vi "ni579x Validate Clock Configuration.vi"(0 "Register Bus":refnum<class "ni579x Register Bus v1 Host.lvclass">=refnum, 1 "scope":string, 5 "clock source":string(combo), 7 "reference clock source":string(combo), 11 "Error In":errorcluster) -> (4 "Register Bus (out)":refnum<class "ni579x Register Bus v1 Host.lvclass">, 6 "coerced clock source":string(combo), 8 "coerced reference clock source":string(combo), 15 "Error Out":errorcluster)   [LabVIEW 2013]
uses:
  <instrlib>/ni579x/Register Bus/v1/Host/ni579x Register Bus v1 Host.lvclass
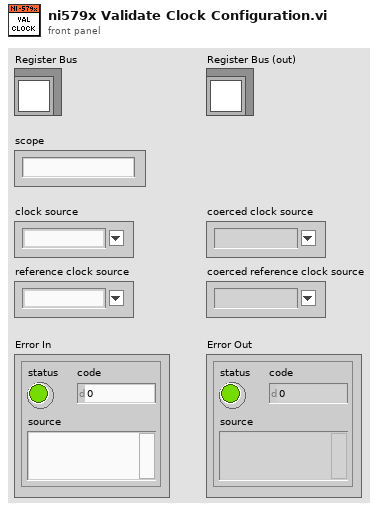
[diagram p1: front panel]
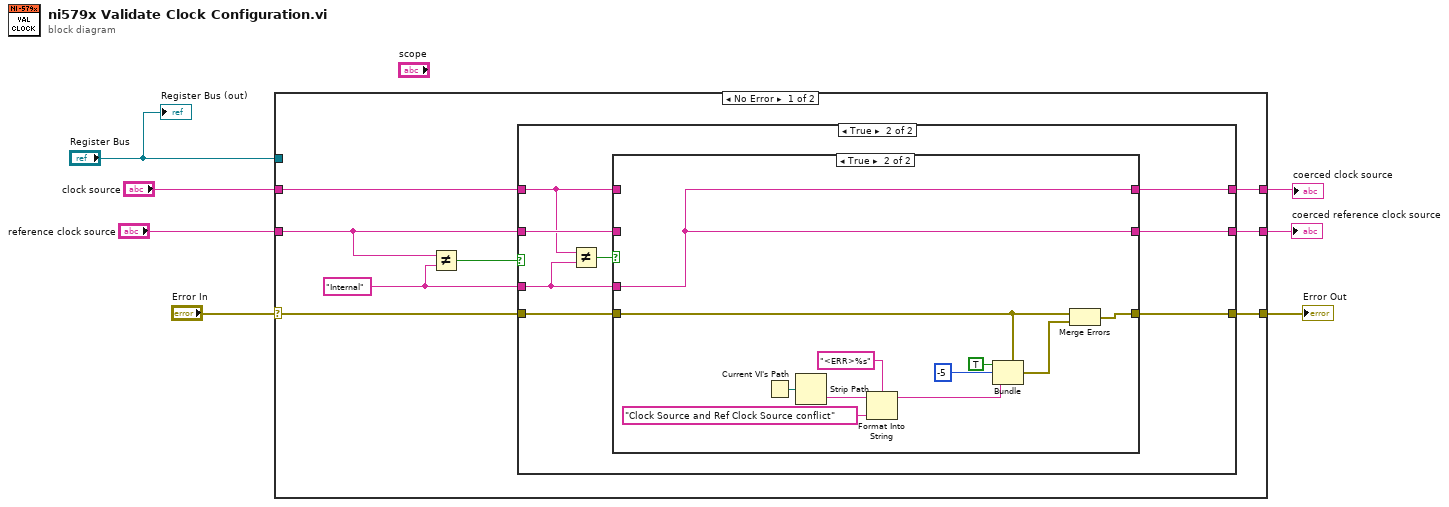
[diagram p0: block diagram]
diagram:
  n1 = case shown="No Error" "Error In" {
    selector: "Error In" -> [w15 w43]
    tunnel: [w14 w43] -> w6
    tunnel: "Register Bus" -> [_ _]
    tunnel: [w11 w42] -> w4
    tunnel: [w10 w41] -> w3
    tunnel: "reference clock source" -> [w9 w41]
    tunnel: "clock source" -> [w8 w42]
    frame No Error {
      w12 = "Internal" ("y")
      n2 = Not Equal?(x=w9, y=w12) -> (x != y?=w13:bool)
      n3 = case shown="True" w13 {
        tunnel: w15 -> [w18 w26]
        tunnel: [w18 w25] -> w14
        tunnel: w8 -> [w17 w22]
        tunnel: w9 -> [w16 w23]
        tunnel: w12 -> [_ w19]
        tunnel: [w17 w21] -> w11
        tunnel: [w16 w20] -> w10
        frame False {
        }
        frame True {
          n4 = Not Equal?(x=w22, y=w19) -> (x != y?=w24:bool)
          n5 = case shown="True" w24 {
            tunnel: w26 -> [w27 w36]
            tunnel: [w27 w34] -> w25
            tunnel: w23 -> [w28 _]
            tunnel: w22 -> [w29 _]
            tunnel: [w29 w30] -> w21
            tunnel: [w28 w30] -> w20
            tunnel: w19 -> [_ w30]
            frame False {
            }
            frame True {
              n6 = Current VI's Path() -> (path=w39:path)
              n7 = Strip Path(path=w39) -> (name=w38:string)  [unwired: 1 out]
              n8 = Format Into String(format string="<ERR>%s", initial string=w38, "Clock Source and Ref Clock Source conflict" ("input 1")) -> (resulting string=w37:string)  [unwired: 1 in, 1 out]
              n9 = Bundle(cluster=w36, "status"=TRUE, "code"=-5, "source"=w37) -> (w35:errorcluster)
              n10 = Merge Errors(w36, w35) -> (w34:errorcluster)
            }
          }
        }
      }
    }
    frame Error {
    }
  }
  "Error Out" <- w6
  "coerced clock source" <- w4
  "coerced reference clock source" <- w3
  "Register Bus (out)" <- "Register Bus"
